vi "FPGA_SICK Write Command.vi"(8 "error in (no error)":errorcluster, 9 "Read/Write Timeout (ms)":i32, 11 "Command index":u32) -> (0 "error out":errorcluster, 1 "Current Command Length":u8, 2 "Timed Out":bool)   [LabVIEW 2009]
uses:
  <vilib>/rvi/DataTransferAndStorage/Container/XNode/niFpgaContainer.xnode
  <vilib>/rvi/Memory/Memory_Emulation/nirvimemoryEmulationManagerCache_GetValue.vi
  <vilib>/rvi/Memory/Memory_Emulation/nirvimemoryEmulationManagerCache_InsertValue.vi
  <vilib>/rvi/DataTransferAndStorage/Container/Common/niFpgaContainerGetUniqueNameForEmu.vi
  <vilib>/Utility/error.llb/Clear Errors.vi
  <vilib>/rvi/Memory/Memory_Emulation/nirvimemoryEmulationManagerCache_SetValue.vi
  <vilib>/eio/EIOMethodNode/EIOMethodNode.xnode
  <vilib>/rvi/eio/nirviEIOMethodImplementation/nirviEIOMethodImplementation.xnode
  <vilib>/rvi/eio/common/nirviEmuTemplateMethod_errors.vi
  <vilib>/rvi/eio/common/nirviEmuClasses.ctl
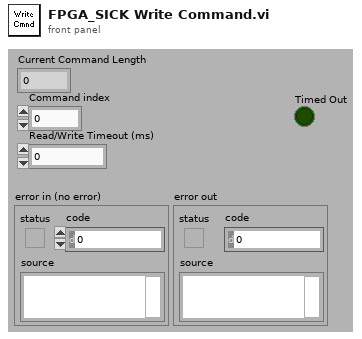
[diagram p1: front panel]
types:
  T1 = typedef "nirviEmuClasses.ctl" = enum16{"IO Read", "IO Write", "Method", "Property Read", "Property Write"}
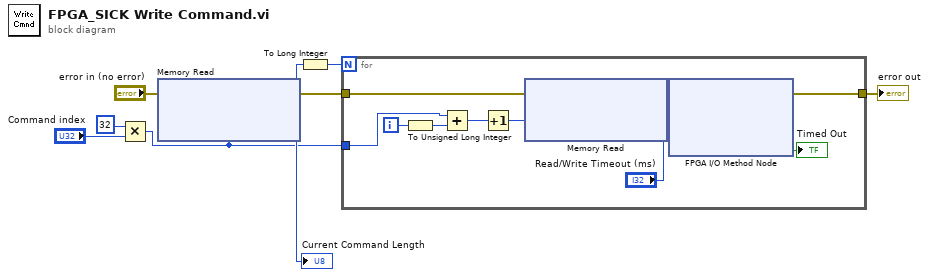
[diagram p0: block diagram]
diagram:
  n1 = Multiply(x=u32 32, y="Command index") -> (x*y=w1:u32)
  n2 = xnode ("Memory Read")("Address"=w1, "error in (no error)"="error in (no error)") -> ("Data"=w5:u8, "error out"=w6:errorcluster)  [unwired: 1 in, 1 out]
  "Current Command Length" <- w5
  n3 = To Long Integer(number=w5) -> (32bit integer=w7:i32)
  n4 = for {
    N: w7 -> [_]
    tunnel: w1 -> [w19]
    tunnel: [w14] -> w2
    tunnel: w6 -> [w13]
    i -> [w18]
    n5 = To Unsigned Long Integer(number=w18) -> (unsigned 32bit integer=w10:u32)
    n6 = Add(x=w19, y=w10) -> (x+y=w16:u32)
    n7 = Increment(x=w16) -> (x+1=w9:u32)
    n8 = xnode ("Memory Read")("Address"=w9, "error in (no error)"=w13) -> ("Data"=w17:u8, "error out"=w15:errorcluster)  [unwired: 1 in, 1 out]
    n9 = xnode "FPGA I/O Method Node"("error in"=w15, "Data"=w17, "Timeout (ms)"="Read/Write Timeout (ms)") -> ("error out"=w14:errorcluster, "Timed Out"=→"Timed Out":bool)  [unwired: 1 in, 1 out]
  }
  "error out" <- w2
